vi "Control-Fuel-Host.vi"() -> ()   [LabVIEW 2016]
uses:
  <vilib>/addons/Software Calibration Management/XControls/TBL2D.xctl
panel:
  out "TempInput":T1 {"Value" format="%#_4p"}
  out "MAPInput":T1 {"Value" format="%#_4p"}
  out "PedalInput":T1 {"Value" format="%#_4p"}
  in  "TempName":string
  in  "MAPName":string
  in  "PedalName":string
  in  "AFR_Stoich":sgl caption="[ratio]" format="%#_4g"
  in  "Fuel_SG":sgl caption="[kg/dm^3]"
  in  "Engine_Vd":sgl caption="[m^3]"
  in  "Lambda_Target":sgl caption="[%]" format="%#_4g"
  out "VE_TblOut":sgl caption="[%]" format="%#_4g"
  in  "TotalFuelQty_Man":sgl caption="[mm3/cyc]"
  in  "Mode":bool
  in  "TotalFuelQty_ManE":bool caption="TotalFuelQty"
  out "TotalFuelQty":sgl caption="[mm3/cyc]" format="%#_4g"
  in  "_TablesTabs":T2(tab)
  in  "TotalFuelQty_Tbl":cluster{"X":sgl[], "Y":sgl[], "Z":sgl[][]}(xcontrol) caption="[Pedal|RPM|mm3/cycle]"
  in  "VE_Tbl":cluster{"X":sgl[], "Y":sgl[], "Z":sgl[][]}(xcontrol) caption="[kPa|RPM|%VE]"
  in  "_Hidden Controls":enum32{"Page 1"}(tab)
  out "Channels|Names":string[](array[string])
  in  "Enable":bool
  # "Engine Fuel Control"
  # "Lambda"
  # "Input Channels"
  # "Channel Name"
  # "Value"
  # "Units"
  # "Pedal (%)"
  # "MAP (kPa)"
  # "MAT (C)"
  # "VE"
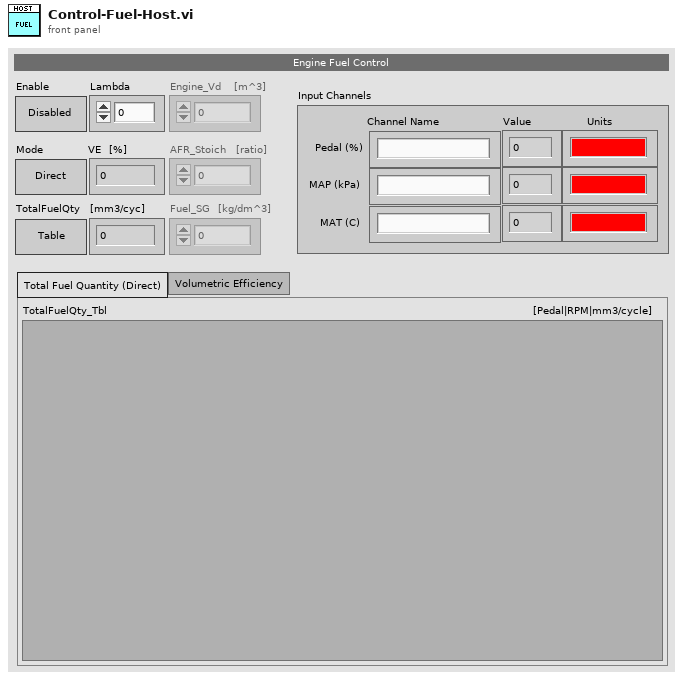
[diagram p1: front panel]
types:
  T1 = cluster{"Name":string, "Unit":string, "Value":sgl}
  T2 = enum32{"Total Fuel Quantity (Direct)", "Volumetric Efficiency"}
  T3 = enum8{"Enabled", "Disabled", "Disabled and Grayed Out"}
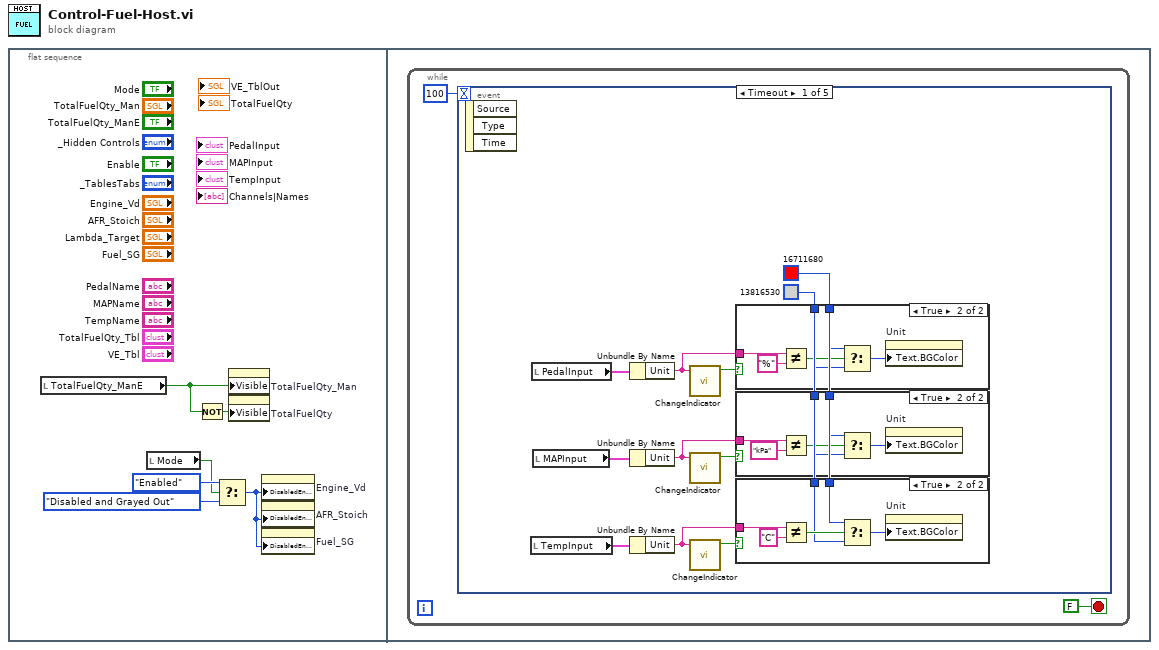
[diagram p0: block diagram]
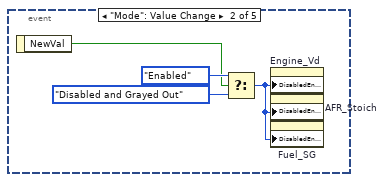
[diagram p5: hidden frame]
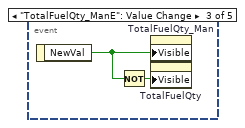
[diagram p6: hidden frame]
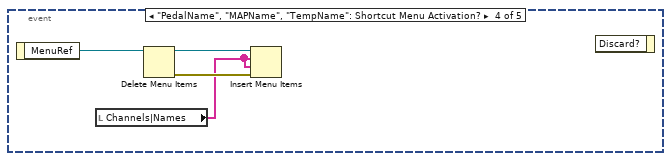
[diagram p7: hidden frame]
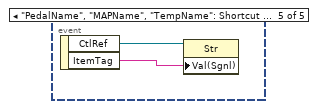
[diagram p8: hidden frame]
diagram:
  n1 = flat-sequence {
    frame #0 {
      n2 = local read "TotalFuelQty_ManE"() -> (w6:bool)
      n3 = local read "Mode"() -> (w2:bool)
      n4 = Not(x=w6) -> (.not. x?=w5:bool)
      n5 = Select(t=T3."Enabled" ("Disabled"), s=w2, f=T3."Disabled and Grayed Out" ("Disabled")) -> (s? t:f=w1:T3)
      n6 = property on="TotalFuelQty_Man" class="DigNum (strict)"("Visible"=w6) -> ()  [unwired: 2 in, 2 out]
      n7 = property on="TotalFuelQty" class="DigNum (strict)"("Visible"=w5) -> ()  [unwired: 2 in, 2 out]
      n8 = property on="Engine_Vd" class="DigNum (strict)"("DisabledEnum"=w1) -> ()  [unwired: 2 in, 2 out]
      n9 = property on="AFR_Stoich" class="DigNum (strict)"("DisabledEnum"=w1) -> ()  [unwired: 2 in, 2 out]
      n10 = property on="Fuel_SG" class="DigNum (strict)"("DisabledEnum"=w1) -> ()  [unwired: 2 in, 2 out]
    }
    frame #1 {
      n11 = while {
        stop <- FALSE stop-if-true
        n12 = event shown="[0] Timeout" {
          selector: _ -> [_ _ _ _ _]
          dyn-events: _ -> [_ _ _ _ _]
          timeout: 100 ("millisecond multiple") -> [_ _ _ _ _]
          event Timeout {
            w9 = u32 16711680 ("Text.Text Colors:BG Color")
            w10 = u32 13816530 ("Text.Text Colors:BG Color")
            n13 = event-data() -> ()  [unwired: 1 in, 3 out]
            n14 = local read "TempInput"() -> (w11:T1)
            n15 = local read "PedalInput"() -> (w17:T1)
            n16 = local read "MAPInput"() -> (w16:T1)
            n17 = Unbundle By Name(w17) -> ("Unit"=w19:string)
            n18 = Unbundle By Name(w16) -> ("Unit"=w14:string)
            n19 = Unbundle By Name(w11) -> ("Unit"=w13:string)
            n20 = call "ChangeIndicator.vi"("Input"=w19) -> ("Change"=w18:bool)  [unwired: 9 in]
            n21 = call "ChangeIndicator.vi"("Input"=w14) -> ("Change"=w15:bool)  [unwired: 9 in]
            n22 = call "ChangeIndicator.vi"("Input"=w13) -> ("Change"=w12:bool)  [unwired: 9 in]
            n23 = case shown="True" w18 {
              tunnel: w19 -> [_ w36]
              tunnel: w9 -> [_ w34]
              tunnel: w10 -> [_ w33]
              frame False {
              }
              frame True {
                n24 = Not Equal?(x=w36, y="%") -> (x != y?=w35:bool)
                n25 = Select(t=w34, s=w35, f=w33) -> (s? t:f=w32:u32)
                n26 = property on="Unit" class="Str"("Text.BGColor"=w32) -> ()  [unwired: 2 in, 2 out]
              }
            }
            n27 = case shown="True" w15 {
              tunnel: w14 -> [_ w30]
              tunnel: w9 -> [_ w28]
              tunnel: w10 -> [_ w27]
              frame False {
              }
              frame True {
                n28 = Not Equal?(x=w30, y="kPa") -> (x != y?=w29:bool)
                n29 = Select(t=w28, s=w29, f=w27) -> (s? t:f=w26:u32)
                n30 = property on="Unit" class="Str"("Text.BGColor"=w26) -> ()  [unwired: 2 in, 2 out]
              }
            }
            n31 = case shown="True" w12 {
              tunnel: w13 -> [_ w24]
              tunnel: w9 -> [_ w22]
              tunnel: w10 -> [_ w21]
              frame False {
              }
              frame True {
                n32 = Not Equal?(x=w24, y="C") -> (x != y?=w23:bool)
                n33 = Select(t=w22, s=w23, f=w21) -> (s? t:f=w20:u32)
                n34 = property on="Unit" class="Str"("Text.BGColor"=w20) -> ()  [unwired: 2 in, 2 out]
              }
            }
          }
          event "Mode": Value Change {
            n35 = event-data() -> ("NewVal"=w39:bool)  [unwired: 1 in]
            n36 = Select(t=T3."Enabled" ("Disabled"), s=w39, f=T3."Disabled and Grayed Out" ("Disabled")) -> (s? t:f=w38:T3)
            n37 = property on="Engine_Vd" class="DigNum (strict)"("DisabledEnum"=w38) -> ()  [unwired: 2 in, 2 out]
            n38 = property on="AFR_Stoich" class="DigNum (strict)"("DisabledEnum"=w38) -> ()  [unwired: 2 in, 2 out]
            n39 = property on="Fuel_SG" class="DigNum (strict)"("DisabledEnum"=w38) -> ()  [unwired: 2 in, 2 out]
          }
          event "TotalFuelQty_ManE": Value Change {
            n40 = event-data() -> ("NewVal"=w42:bool)  [unwired: 1 in]
            n41 = Not(x=w42) -> (.not. x?=w43:bool)
            n42 = property on="TotalFuelQty_Man" class="DigNum (strict)"("Visible"=w42) -> ()  [unwired: 2 in, 2 out]
            n43 = property on="TotalFuelQty" class="DigNum (strict)"("Visible"=w43) -> ()  [unwired: 2 in, 2 out]
          }
          event "PedalName", "MAPName", "TempName": Shortcut Menu Activation? {
            n44 = event-data() -> ("MenuRef"=w47:refnum<k9>)  [unwired: 1 in]
            n45 = local read "Channels|Names"() -> (w44:string[])
            n46 = Delete Menu Items(9:w47) -> (0:w45:errorcluster, 3:w46:refnum<k9>)  [unwired: 3 in]
            n47 = Insert Menu Items(6:w45, 7:w44, 8:w44, 9:w46) -> ()  [unwired: 2 in, 3 out]
            n48 = event-data() -> ()  [unwired: 2 in, 1 out]
          }
          event "PedalName", "MAPName", "TempName": Shortcut Menu Selection (User) {
            n49 = event-data() -> ("CtlRef"=w49:refnum<vi>, "ItemTag"=w48:string)  [unwired: 1 in]
            n50 = property class="Str"(reference=w49, "Val(Sgnl)"=w48) -> ()  [unwired: 1 in, 2 out]
          }
        }
      }
    }
  }
